vi "SN Report Number Increase.vi"(9 "Sample #":string="151600001", 10 "Report No.":string="HF-151600001", 11 "S/N:":string="151600001") -> (1 "Sample # out":string="151600001", 2 "Report No. out":string="HF-151600001", 3 "S/N_out":string="151600001" caption="S/N:")   [LabVIEW 2011]
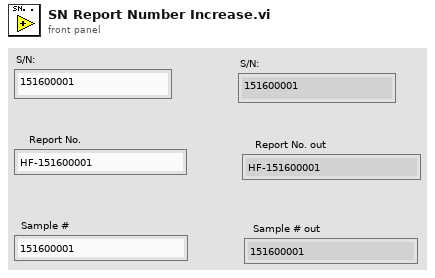
[diagram p1: front panel]
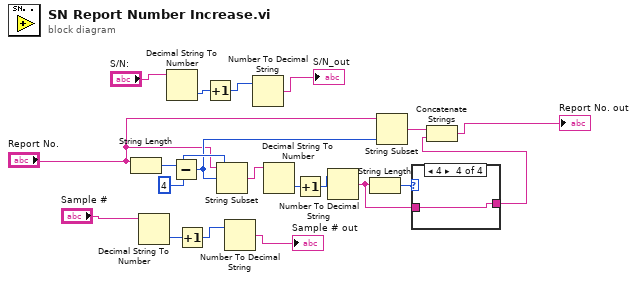
[diagram p0: block diagram]
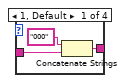
[diagram p2: hidden frame]
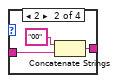
[diagram p3: hidden frame]
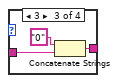
[diagram p4: hidden frame]
diagram:
  w15 = 4 ("长度（剩余）")
  n1 = String Length(string="Report No.") -> (length=w16:i32)
  n2 = Decimal String To Number(string="Sample #") -> (number=w17:i32)  [unwired: 2 in, 1 out]
  n3 = Decimal String To Number(string="S/N:") -> (number=w20:i32)  [unwired: 2 in, 1 out]
  n4 = Subtract(x=w16, y=w15) -> (x-y=w11:i32)
  n5 = Increment(x=w17) -> (x+1=w18:i32)
  n6 = Increment(x=w20) -> (x+1=w19:i32)
  n7 = String Subset(string="Report No.", offset (0)=w11, length (rest)=w15) -> (substring=w14:string)
  n8 = Number To Decimal String(number=w18) -> (decimal integer string=→"Sample # out":string)  [unwired: 1 in]
  n9 = Number To Decimal String(number=w19) -> (decimal integer string=→"S/N_out":string)  [unwired: 1 in]
  n10 = Decimal String To Number(string=w14) -> (number=w13:i32)  [unwired: 2 in, 1 out]
  n11 = Increment(x=w13) -> (x+1=w12:i32)
  n12 = Number To Decimal String(number=w12) -> (decimal integer string=w8:string)  [unwired: 1 in]
  n13 = String Length(string=w8) -> (length=w9:i32)
  n14 = String Subset(string="Report No.", length (rest)=w11) -> (substring=w10:string)  [unwired: 1 in]
  n15 = case shown="4" w9 {
    tunnel: w8 -> [w23 w26 w29 w30]
    tunnel: [w21 w24 w27 w30] -> w7
    frame 1, Default {
      n16 = Concatenate Strings("000" ("字符串"), w23) -> (w21:string)
    }
    frame 2 {
      n17 = Concatenate Strings("00" ("字符串"), w26) -> (w24:string)
    }
    frame 3 {
      n18 = Concatenate Strings("0" ("字符串"), w29) -> (w27:string)
    }
    frame 4 {
    }
  }
  n19 = Concatenate Strings(w10, w7) -> (→"Report No. out":string)
